vi "build_T1_curve.vi"(8 "T1_parameters":T1, 9 "timetags":u32[][](array[numeric]), 10 "stop_read":u32[][](array[numeric]), 11 "start_read":u32[][](array[numeric])) -> (1 "histogram":cluster{"q_photons":i32[], "histogram":i32[]}, 2 "T1 curve":cluster{"dark_time_us":dbl[], "PL_signal":i32[]}, 3 "error_bars":cluster{"dark_times_us":dbl[], "error":dbl[]})   [LabVIEW 2018]
uses:
  <vilib>/Analysis/NI_AALBase.lvlib
panel:
  out "photons_counts":i32[][](array[numeric])
  out "std_deviation":dbl[](array[numeric])
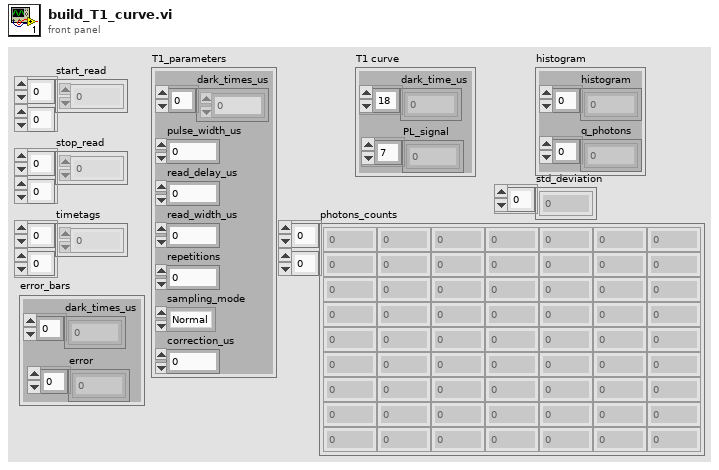
[diagram p1: front panel]
types:
  T1 = cluster{"dark_times_us":dbl[], "pulse_width_us":dbl, "read_delay_us":dbl, "read_width_us":dbl, "repetitions":i32, "sampling_mode":enum16{"Normal", "Sweep"}, "correction_us":dbl}
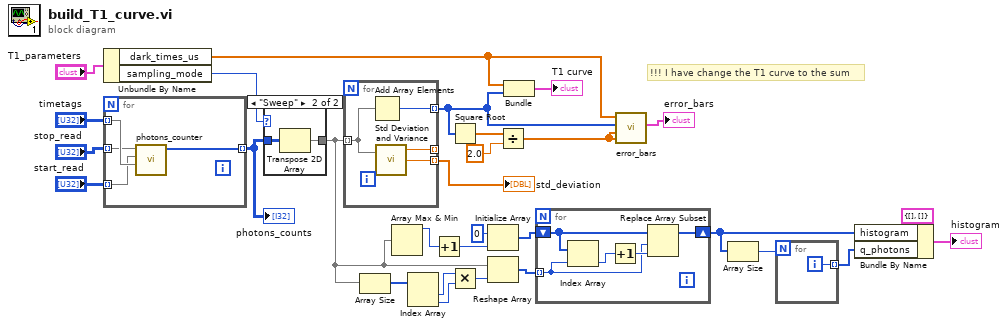
[diagram p0: block diagram]
diagram:
  # "!!! I have change the T1 curve to the sum"
  n1 = Unbundle By Name("T1_parameters") -> ("dark_times_us"=w1:dbl[], "sampling_mode"=w21:enum16{"Normal", "Sweep"})
  n2 = for {
    tunnel: "timetags" -> [w33] mode=indexing
    tunnel: "stop_read" -> [w32] mode=indexing
    tunnel: "start_read" -> [w31] mode=indexing
    tunnel: [w30] -> w27 mode=indexing
    n3 = call "photons_counter.vi"("timetags"=w33, "start_read"=w31, "stop_read"=w32) -> ("photons_counts"=w30:i32[])  [unwired: 8 in]
  }
  "photons_counts" <- w27
  n4 = case shown="\"Sweep\"" w21 {
    tunnel: w27 -> [w34 w36]
    tunnel: [w34 w35] -> w17
    frame "Normal", Default {
    }
    frame "Sweep" {
      n5 = Transpose 2D Array(2D array=w36) -> (transposed array=w35:i32[][])
    }
  }
  n6 = for {
    tunnel: w17 -> [w38] mode=indexing
    tunnel: [w40] -> _ mode=indexing
    tunnel: [w39] -> w6 mode=indexing
    tunnel: [w37] -> w2 mode=indexing
    n7 = Add Array Elements(numeric array=w38) -> (sum=w37:i32)
    n8 = call <vilib>:"Std Deviation and Variance.vi"("X"=w38) -> ("mean"=w40:dbl, "standard deviation"=w39:dbl)  [unwired: 1 in, 1 out]
  }
  "std_deviation" <- w6
  n9 = Array Size(array=w17) -> (size(s)=w25:i32[])
  n10 = Array Max & Min(array=w17) -> (max value=w20:i32)  [unwired: 3 out]
  n11 = Index Array(array=w25) -> (element #1=w22:i32, element #2=w24:i32)  [unwired: 2 in]
  n12 = Increment(x=w20) -> (x+1=w15:i32)
  n13 = Square Root(x=w2) -> (sqrt(x)=w5:dbl[])
  n14 = Multiply(x=w22, y=w24) -> (x*y=w23:i32)
  n15 = Initialize Array(0 ("element"), w15) -> (w16:i32[])
  n16 = Reshape Array(w17, w23) -> (w18:i32[])
  n17 = Divide(x=w5, y=2.0) -> (x/y=w3:dbl[])
  n18 = Bundle("dark_times_us"=w1, w2) -> (→"T1 curve":cluster{"dark_times_us":dbl[], i32[]})  [unwired: 1 in]
  n19 = for {
    tunnel: w18 -> [w42] mode=indexing
    shift-right: [w44] -> w12
    shift-left: w16 -> [w43]
    n20 = Index Array(array=w43, index=w42) -> (element=w41:i32)
    n21 = Increment(x=w41) -> (x+1=w45:i32)
    n22 = Replace Array Subset(array=w43, new element=w45, index=w42) -> (w44:i32[])
  }
  n23 = call "error_bars.vi"("y_error-"=w3, "y_error+"=w3, "y"=w2, "x"=w1) -> ("error_bars"=→"error_bars":cluster{"dark_times_us":dbl[], dbl[]})  [unwired: 7 in]
  n24 = Array Size(array=w12) -> (size(s)=w14:i32)
  n25 = for {
    N: w14 -> [_]
    tunnel: [w46] -> w11 mode=indexing
    i -> [w46]
  }
  n26 = Bundle By Name(cluster=cluster{"q_photons":i32[], "histogram":i32[]} {"q_photons"=[], "histogram"=[]} ("histogram"), "histogram"=w12, "q_photons"=w11) -> (→"histogram":cluster{"q_photons":i32[], "histogram":i32[]})
